vi "spektrum.vi"(11 "wykres 1":waveform(dbl)) -> (1 "df":dbl, 2 "As z A(1)":cdb[](array[numeric]), 3 "As":cdb[](array[numeric]), 4 "wykres 2":waveform(dbl), 5 "N2":dbl)   [LabVIEW 2025]
uses:
  <vilib>/Analysis/2dsp.llb/Real FFT.vi
  <vilib>/Analysis/NI_AALPro.lvlib
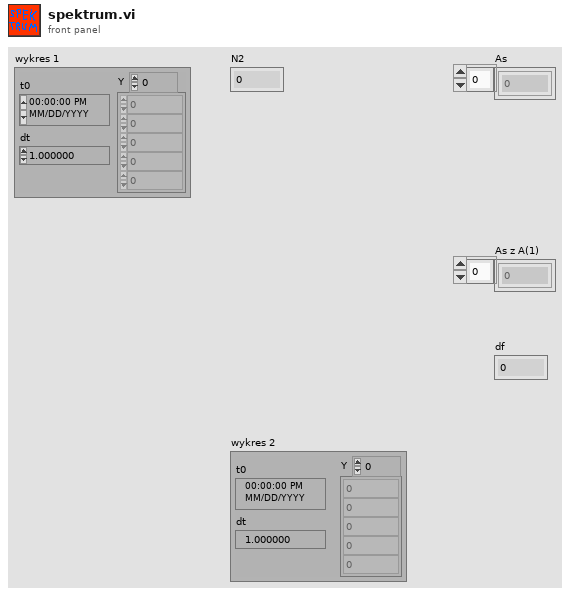
[diagram p1: front panel]
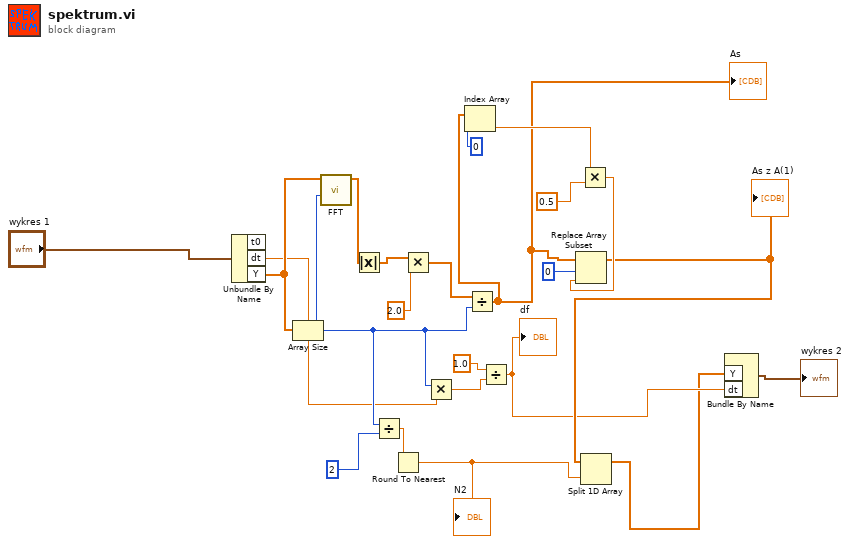
[diagram p0: block diagram]
diagram:
  n1 = Unbundle By Name("wykres 1") -> ("dt"=w7:dbl, "Y"=w23:dbl[])  [unwired: 1 out]
  n2 = Array Size(array=w23) -> (size(s)=w18:i32)
  n3 = call-poly <vilib>:"FFT.vi"("FFT size"=w18, "X"=w23) -> ("FFT {X}"=w10:cdb[])  [unwired: 8 in, 1 out]
  n4 = Absolute Value(x=w10) -> (abs(x)=w9:dbl[])
  n5 = Divide(x=w18, y=2) -> (x/y=w16:dbl)
  n6 = Round To Nearest(number=w16) -> (nearest integer value=w5:dbl)
  "N2" <- w5
  n7 = Multiply(x=w9, y=2.0) -> (x*y=w21:dbl[])
  n8 = Multiply(x=w18, y=w7) -> (x*y=w19:dbl)
  n9 = Divide(x=w21, y=w18) -> (x/y=w11:dbl[])
  "As" <- w11
  n10 = Index Array(array=w11, index=0) -> (element=w13:dbl)
  n11 = Divide(x=1.0, y=w19) -> (x/y=w3:dbl)
  "df" <- w3
  n12 = Multiply(x=w13, y=0.5) -> (x*y=w12:dbl)
  n13 = Replace Array Subset(array=w11, new element=w12, index=0) -> (w6:dbl[])
  "As z A(1)" <- w6
  n14 = Split 1D Array(array=w6, index=w5) -> (first subarray=w2:dbl[])  [unwired: 1 out]
  n15 = Bundle By Name("Y"=w2, "dt"=w3) -> (→"wykres 2":waveform(dbl))  [unwired: 1 in]
